vi "Get Server URL.vi"(11 "DeepL Free API?":bool) -> (3 "url":string)   [LabVIEW 2015, in "lv-deepl-api.lvlib"]
uses:
  lv-deepl-api.lvlib
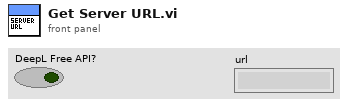
[diagram p1: front panel]
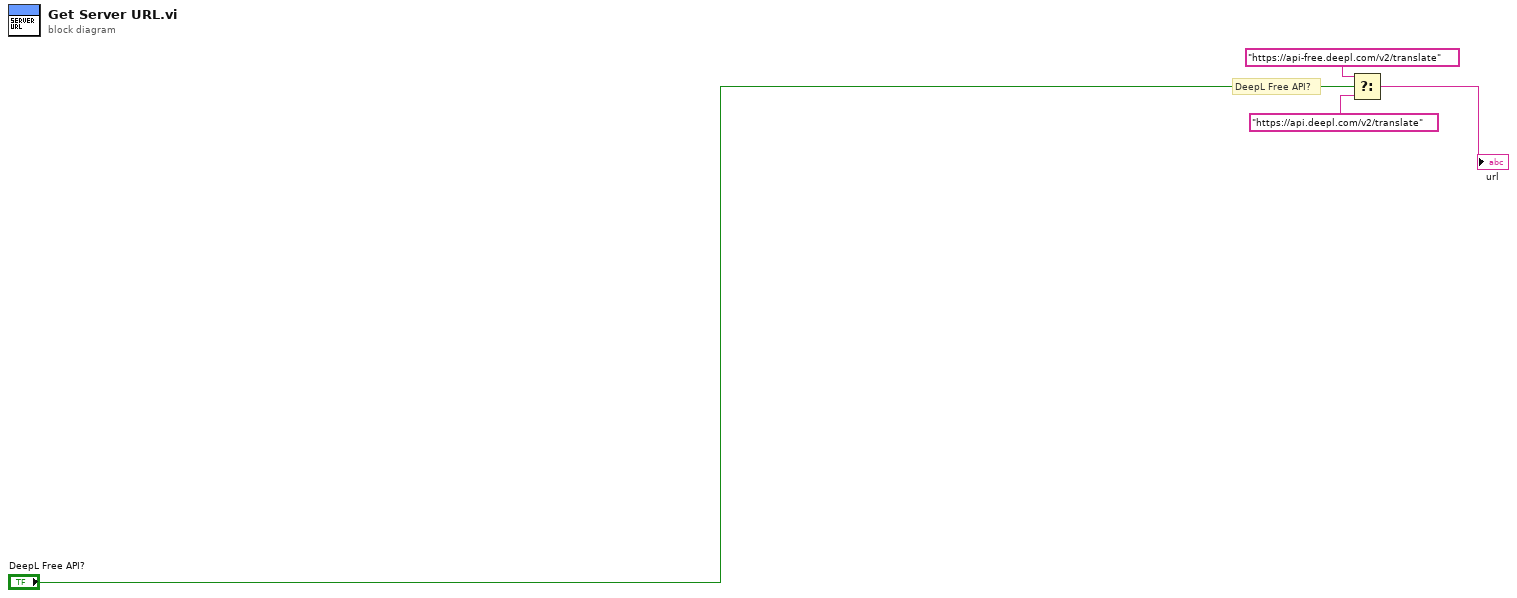
[diagram p0: block diagram]
diagram:
  # "DeepL Free API?"
  n1 = Select(t="https://api-free.deepl.com/v2/translate" ("url"), s="DeepL Free API?", f="https://api.deepl.com/v2/translate" ("url")) -> (s? t:f=→"url":string)
